vi "SP Convert Frequency from MHz.vi"(7 "Sweep":T2={"Fstart"=-1.0, "Fstop"=-1.0, "Units"=enum."Hz", "Points"=-1}, 10 "Units":T1=enum."MHz", 11 "Frequency (MHz)":dbl) -> (3 "Converted Frequency":dbl)   [LabVIEW 2011]
uses:
  TypeDefs/SP Frequency Units.ctl
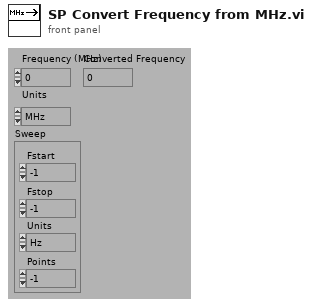
[diagram p1: front panel]
types:
  T1 = typedef "SP Frequency Units.ctl" = enum16{"Hz", "kHz", "MHz", "GHz", "Points"}
  T2 = cluster{"Fstart":dbl, "Fstop":dbl, "Units":T1, "Points":i32}
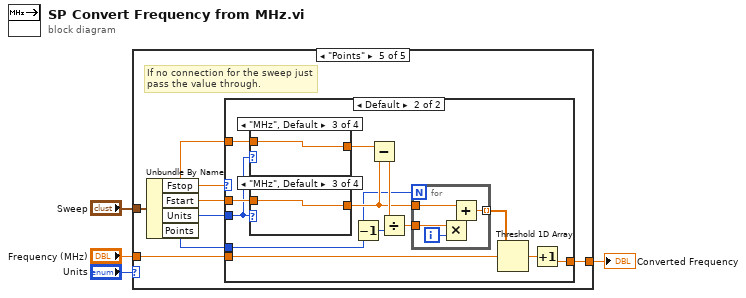
[diagram p0: block diagram]
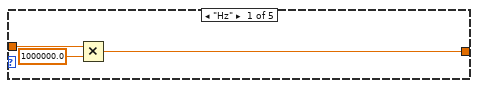
[diagram p2: hidden frame]
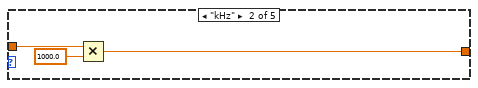
[diagram p3: hidden frame]
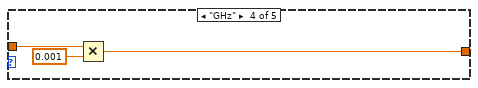
[diagram p5: hidden frame]
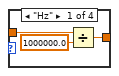
[diagram p7: hidden frame]
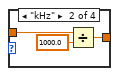
[diagram p8: hidden frame]
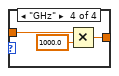
[diagram p9: hidden frame]
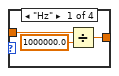
[diagram p10: hidden frame]
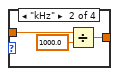
[diagram p11: hidden frame]
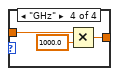
[diagram p12: hidden frame]
diagram:
  n1 = case shown="\"Points\"" "Units" {
    tunnel: "Frequency (MHz)" -> [w7 w10 w11 w14 w21]
    tunnel: [w6 w9 w11 w13 w19] -> w4
    tunnel: "Sweep" -> [_ _ _ _ w20]
    frame "Hz" {
      n2 = Multiply(x=w7, y=1000000.0) -> (x*y=w6:dbl)
    }
    frame "kHz" {
      n3 = Multiply(x=w10, y=1000.0) -> (x*y=w9:dbl)
    }
    frame "MHz" {
    }
    frame "GHz" {
      n4 = Multiply(x=w14, y=0.001) -> (x*y=w13:dbl)
    }
    frame "Points" {
      # "If no connection for the sweep just\npass the value through."
      n5 = Unbundle By Name(w20) -> ("Fstop"=w15:dbl, "Fstart"=w18:dbl, "Units"=w17:T1, "Points"=w16:i32)
      n6 = case shown="Default" w15 {
        tunnel: w21 -> [w22 w24]
        tunnel: [w22 w25] -> w19
        tunnel: w15 -> [_ w35]
        tunnel: w18 -> [_ w34]
        tunnel: w17 -> [_ w33]
        tunnel: w16 -> [_ w23]
        frame -1 {
        }
        frame Default {
          n7 = case shown="\"MHz\", Default" w33 {
            tunnel: w35 -> [w53 w55 w57 w60]
            tunnel: [w52 w54 w57 w59] -> w27
            frame "Hz" {
              n8 = Divide(x=w53, y=1000000.0) -> (x/y=w52:dbl)
            }
            frame "kHz" {
              n9 = Divide(x=w55, y=1000.0) -> (x/y=w54:dbl)
            }
            frame "MHz", Default {
            }
            frame "GHz" {
              n10 = Multiply(x=w60, y=1000.0) -> (x*y=w59:dbl)
            }
          }
          n11 = case shown="\"MHz\", Default" w33 {
            tunnel: w34 -> [w43 w45 w47 w50]
            tunnel: [w42 w44 w47 w49] -> w26
            frame "Hz" {
              n12 = Divide(x=w43, y=1000000.0) -> (x/y=w42:dbl)
            }
            frame "kHz" {
              n13 = Divide(x=w45, y=1000.0) -> (x/y=w44:dbl)
            }
            frame "MHz", Default {
            }
            frame "GHz" {
              n14 = Multiply(x=w50, y=1000.0) -> (x*y=w49:dbl)
            }
          }
          n15 = Decrement(x=w23) -> (x-1=w32:i32)
          n16 = Subtract(x=w27, y=w26) -> (x-y=w28:dbl)
          n17 = Divide(x=w28, y=w32) -> (x/y=w29:dbl)
          n18 = for {
            N: w23 -> [_]
            tunnel: w26 -> [w40]
            tunnel: w29 -> [w39]
            tunnel: [w36] -> w30 mode=indexing
            i -> [w38]
            n19 = Multiply(x=w39, y=w38) -> (x*y=w37:dbl)
            n20 = Add(x=w40, y=w37) -> (x+y=w36:dbl)
          }
          n21 = Threshold 1D Array(2:w24, 3:w30) -> (0:w31:dbl)  [unwired: 1 out]
          n22 = Increment(x=w31) -> (x+1=w25:dbl)
        }
      }
    }
  }
  "Converted Frequency" <- w4
